vi "Drive Train Task.vi"(8 "Period":i64, 10 "Match Info":T1={"Autonomous Elapsed Seconds"=0.0, "TeleOp Elapsed Seconds"=0.0, "Disabled Elapsed Seconds"=0.0, "Visited Autonomous"=FALSE, "Visited TeleOp"=FALSE, "Visited Disabled"=FALSE, "Autonomous Settings"={"Autonomous Style"=enum."Independent", "VI Refnum"=refnum}}, 11 "Refnum in":refnum<k33>) -> ()   [LabVIEW 2014]
uses:
  <vilib>/Rock Robotics/WPI/DriverStation/WPI_DriverStationMatch Info.ctl
  TeleopCmd.ctl
  CmdFlag.ctl
  Drive Train States.ctl
  Drive Train Metrics.ctl
  <vilib>/Platform/TimedLoop/XDataNode/timing_clust.ctl
  <vilib>/Platform/TimedLoop/XDataNode/nitl_modes.ctl
  <vilib>/Platform/TimedLoop/XDataNode/wakeup.ctl
  <vilib>/platform/TimedLoop/XDataNode/XDataNode.xnode
  <vilib>/Platform/TimedLoop/XDataNode/XDNodeRunTimeDep.lvlib
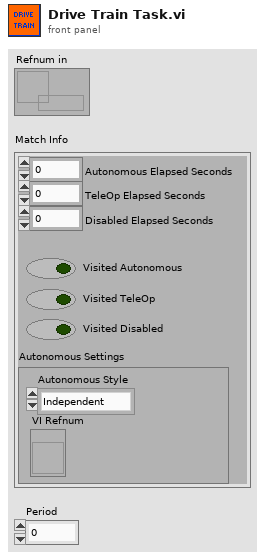
[diagram p1: front panel]
types:
  T1 = typedef "WPI_DriverStationMatch Info.ctl" = cluster{"Autonomous Elapsed Seconds":dbl, "TeleOp Elapsed Seconds":dbl, "Disabled Elapsed Seconds":dbl, "Visited Autonomous":bool, "Visited TeleOp":bool, "Visited Disabled":bool, "Autonomous Settings":cluster{"Autonomous Style":enum16{"Iterative", "Independent"}, "VI Refnum":refnum<vi>}}
  T2 = typedef "Drive Train Metrics.ctl" = cluster{"last time in gear":u32, "Shift":bool, "Right Joystick":dbl, "Left Joystick":dbl, "CmdFlag":T3, "Right Motor Power":dbl, "Left Motor Power":dbl, "Right Accel.":dbl, "Left Accel.":dbl, "Filtered Left Drive Rate":dbl, "Filtered Right Drive Rate":dbl, "Direction of travel":enum16{"Backward", "Forward", "Spin"}, "AverageAccelleration":dbl, "Time of Last Metric":u32, "Time Of Last Shift":dbl, "Average Drive Rate":dbl, "Average Throttle":dbl, "FIFO Timeout":i32, "Requested Left Velocity":dbl, "Requested Right Velocity":dbl}
  T3 = typedef "CmdFlag.ctl" = enum16{"noop", "suspend", "resume"}
  T4 = typedef "Drive Train States.ctl" = enum16{"Auton", "Initialize", "Drive", "Suspend", "Resume"}
  T5 = typedef "XDNodeRunTimeDep.lvlib/timing_clust.ctl" = cluster{"Expected End [f-1]":u64, "Actual End [f-1]":u64, "Finished Late? [f-1]":bool, "Expected End [i-1]":u64, "Actual End [i-1]":u64, "Finished Late? [i-1]":bool, "Expected Start [i]":u64, "Actual Start [i]":u64, "Expected Start [f]":u64, "Actual Start [f]":u64, "Source Name":string, "Structure Name":string, "Period":i64, "Deadline":i64, "Offset":i64, "Start":i64, "Priority":i32, "Timeout":i32, "Mode":T6, "Wakeup Reason":T7, "Error":errorcluster, "Source Type":string, "Secondary Source Type":string, "Global End Time":u64, "Global Start Time":u64, "Frame Duration":u64, "Iteration Duration":u64, "Assigned CPU":i32, "I/O Scan Engine Mode":u32}
  T6 = typedef "XDNodeRunTimeDep.lvlib/nitl_modes.ctl" = enum32{"No Change", "Process missed periods, maintain original phase", "Discard missed periods, maintain original phase", "Process missed periods, ignore original phase", "Discard missed periods, ignore original phase"}
  T7 = typedef "XDNodeRunTimeDep.lvlib/wakeup.ctl" = enum32{"Normal", "Aborted", "Asynchronous wakeup", "Timing source error", "Timed loop error", "Timeout"}
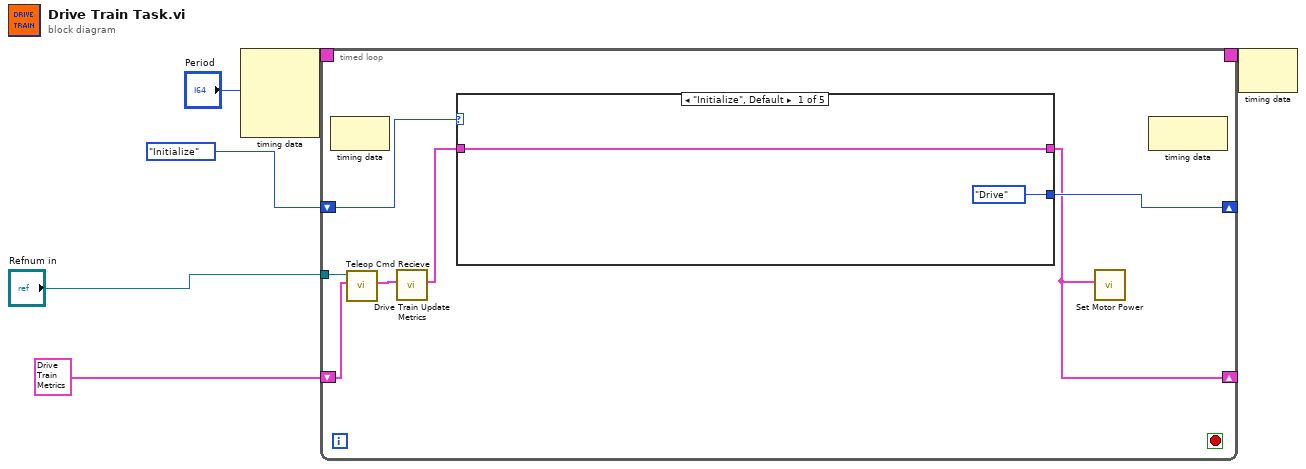
[diagram p0: block diagram]
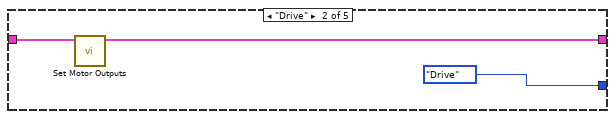
[diagram p2: hidden frame]
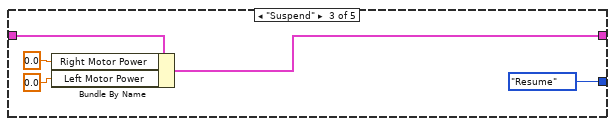
[diagram p3: hidden frame]
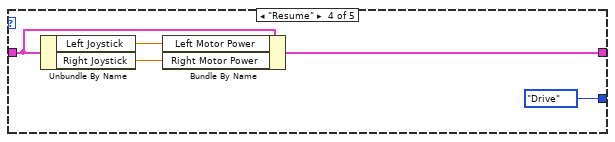
[diagram p4: hidden frame]
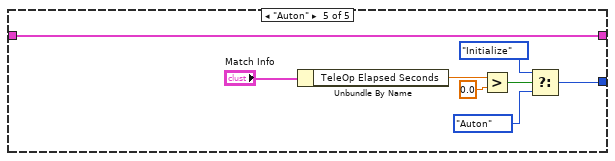
[diagram p5: hidden frame]
diagram:
  n1 = node-c288("Period") -> (w6:T5)  [unwired: 3 in]
  n2 = timed-loop {
    timing: w6 -> [_]
    timing-out: [_] -> w5
    tunnel: "Refnum in" -> [w13]
    shift-right: [w10] -> _
    shift-left: Drive_Train_States."Initialize" ("Enum") -> [w11]
    shift-right: [w8] -> _
    shift-left: T2 {"last time in gear"=0, "Shift"=FALSE, "Right Joystick"=0.0, "Left Joystick"=0.0, "CmdFlag"=enum."noop", "Right Motor Power"=0.0, "Left Motor Power"=0.0, "Right Accel."=0.0, "Left Accel."=0.0, "Filtered Left Drive Rate"=0.0, "Filtered Right Drive Rate"=0.0, "Direction of travel"=enum."Backward", "AverageAccelleration"=0.0, "Time of Last Metric"=0, "Time Of Last Shift"=0.0, "Average Drive Rate"=0.0, "Average Throttle"=0.0, "FIFO Timeout"=0, "Requested Left Velocity"=0.0, "Requested Right Velocity"=0.0} ("Cluster") -> [w12]
    stop <- _ stop-if-true
    n3 = node-c288() -> ()  [unwired: 1 in, 1 out]
    n4 = call "Teleop Cmd Recieve.vi"("Metrics Input"=w12, "rt fifo"=w13) -> ("Updated Drive Metrics"=w7:T2)  [unwired: 8 in, 1 out]
    n5 = call "Drive Train Update Metrics.vi"("Input"=w7) -> ("Output"=w9:T2)  [unwired: 10 in]
    n6 = case shown="\"Initialize\", Default" w11 {
      tunnel: [Drive_Train_States."Drive" ("Enum") Drive_Train_States."Drive" ("Enum") Drive_Train_States."Resume" ("Enum") Drive_Train_States."Drive" ("Enum") w34] -> w10
      tunnel: w9 -> [w14 w17 w22 w24 w29]
      tunnel: [w14 w16 w19 w25 w29] -> w8
      frame "Initialize", Default {
      }
      frame "Drive" {
        n7 = call "Set Motor Outputs.vi"("Updated Drive Metrics in"=w17) -> ("Updated Drive Metrics out"=w16:T2)  [unwired: 10 in]
      }
      frame "Suspend" {
        n8 = Bundle By Name(cluster=w22, "Right Motor Power"=0.0, "Left Motor Power"=0.0) -> (w19:T2)
      }
      frame "Resume" {
        n9 = Unbundle By Name(w24) -> ("Left Joystick"=w27:dbl, "Right Joystick"=w26:dbl)
        n10 = Bundle By Name(cluster=w24, "Left Motor Power"=w27, "Right Motor Power"=w26) -> (w25:T2)
      }
      frame "Auton" {
        n11 = Unbundle By Name("Match Info") -> ("TeleOp Elapsed Seconds"=w32:dbl)
        n12 = Greater?(x=w32, y=0.0) -> (0:w30:bool)
        n13 = Select(t=Drive_Train_States."Initialize" ("Enum"), s=w30, f=Drive_Train_States."Auton" ("Enum")) -> (s? t:f=w34:T4)
      }
    }
    n14 = call "Set Motor Power.vi"("Cluster"=w8) -> ()  [unwired: 11 in]
    n15 = node-c288() -> ()  [unwired: 1 in, 1 out]
  }
  n16 = node-c288(w5) -> ()  [unwired: 1 out]
